vi "Find Packed Libraries.vi"(8 "error in (no error)":errorcluster, 11 "Component Loader in":refnum<class "Component Loader.lvclass">) -> (0 "error out":errorcluster, 2 "packed library paths":path[](array[path]), 3 "Component Loader out":refnum<class "Component Loader.lvclass">)   [LabVIEW 2017, in "Data Sharing Framework Engine.lvlib" / "Component Loader.lvclass"]
uses:
  Component Loader.lvclass
  Component Loader.lvclass/Component Loader.ctl
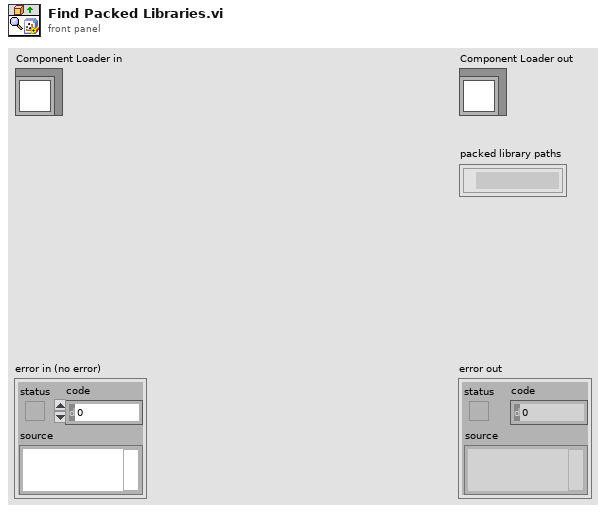
[diagram p1: front panel]
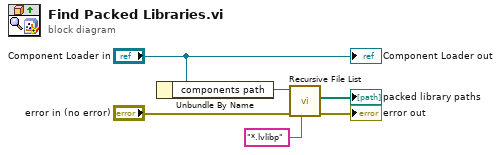
[diagram p0: block diagram]
diagram:
  n1 = Unbundle By Name("Component Loader in") -> ("components path"=w2:path)
  n2 = call <vilib>:"Recursive File List.vi"("pattern"="*.lvlibp", "error in (no error)"="error in (no error)", "Folder Path"=w2) -> ("error out"=→"error out":errorcluster, "All Files in Dir"=→"packed library paths":path[])  [unwired: 4 in, 3 out]
  "Component Loader out" <- "Component Loader in"
